vi "Network Error Core.vi"(8 "error in (no error)":errorcluster, 10 "String to Append":string, 11 "Error":T1) -> (0 "error out":errorcluster)   [LabVIEW 2021, in "Networking_CIF_U.lvlib"]
uses:
  Networking_CIF_U.lvlib
  Typedef/Errors.ctl
  Errors/Errors_CIF_U.lvlib
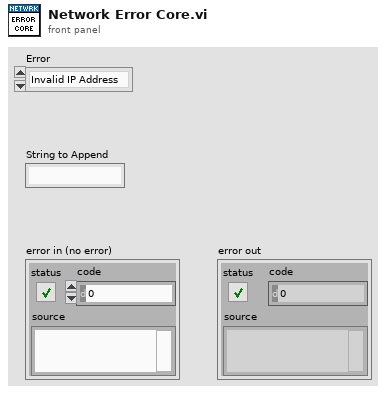
[diagram p1: front panel]
types:
  T1 = typedef "Networking_CIF_U.lvlib/Errors.ctl" = enum16{"Invalid IP Address", "No Subnet Match Found", "Error Finding Port", "No Ping Response", "Nettools Needed", "Error Checking Port"}
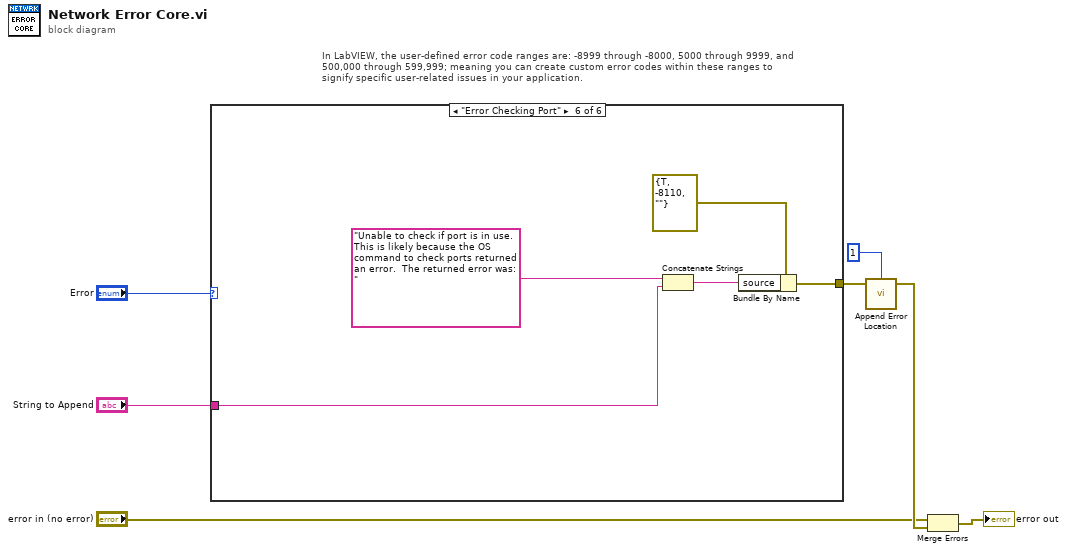
[diagram p0: block diagram]
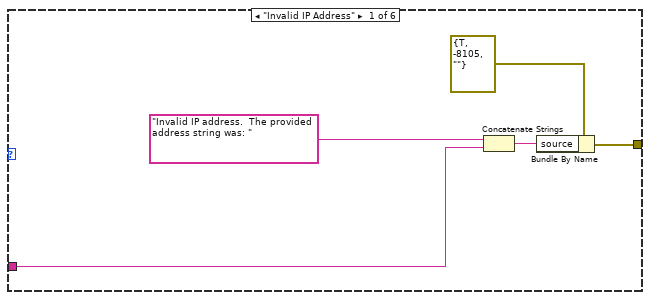
[diagram p2: hidden frame]
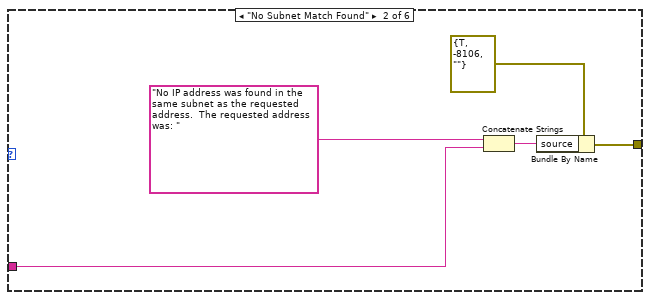
[diagram p3: hidden frame]
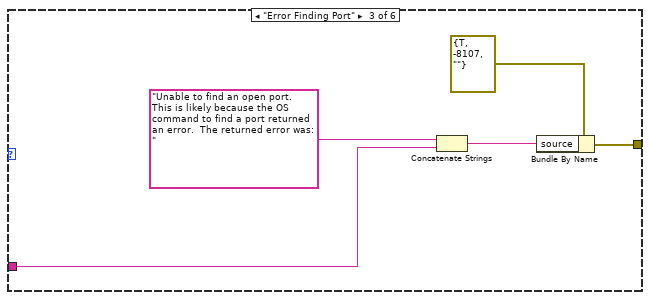
[diagram p4: hidden frame]
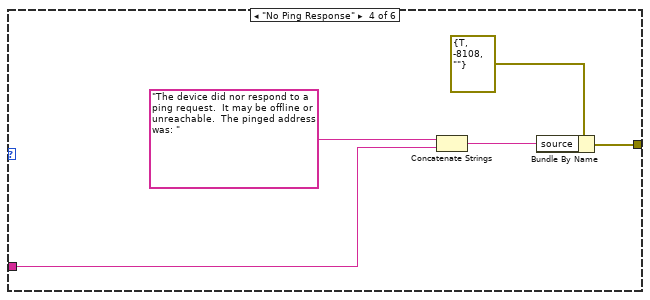
[diagram p5: hidden frame]
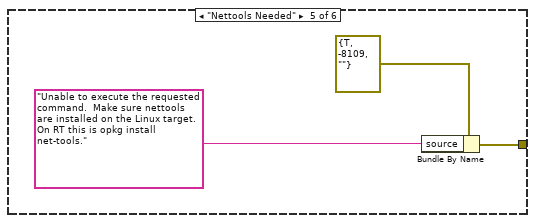
[diagram p6: hidden frame]
diagram:
  # "In LabVIEW, the user-defined error code ranges are: -8999 through -8000, 5000 through 9999, and 500,000 through 599,999; meaning you can create custom error codes within these ranges to signify specific user-related issues in your application."
  n1 = case shown="\"Error Checking Port\"" "Error" {
    tunnel: "String to Append" -> [w9 w14 w18 w23 _ w31]
    tunnel: [w11 w16 w21 w26 w29 w34] -> w6
    frame "Invalid IP Address" {
      n2 = Concatenate Strings("Invalid IP address.  The provided address string was: " ("source"), w9) -> (w8:string)
      n3 = Bundle By Name(cluster=errorcluster {"status"=TRUE, "code"=-8105, "source"=""} ("Invalid ID"), "source"=w8) -> (w11:errorcluster)
    }
    frame "No Subnet Match Found" {
      n4 = Concatenate Strings("No IP address was found in the same subnet as the requested address.  The requested address was: " ("source"), w14) -> (w13:string)
      n5 = Bundle By Name(cluster=errorcluster {"status"=TRUE, "code"=-8106, "source"=""} ("Invalid ID"), "source"=w13) -> (w16:errorcluster)
    }
    frame "Error Finding Port" {
      n6 = Concatenate Strings("Unable to find an open port.  This is likely because the OS command to find a port returned an error.  The returned error was: " ("source"), w18) -> (w19:string)
      n7 = Bundle By Name(cluster=errorcluster {"status"=TRUE, "code"=-8107, "source"=""} ("Invalid ID"), "source"=w19) -> (w21:errorcluster)
    }
    frame "No Ping Response" {
      n8 = Concatenate Strings("The device did nor respond to a ping request.  It may be offline or unreachable.  The pinged address was: " ("source"), w23) -> (w24:string)
      n9 = Bundle By Name(cluster=errorcluster {"status"=TRUE, "code"=-8108, "source"=""} ("Invalid ID"), "source"=w24) -> (w26:errorcluster)
    }
    frame "Nettools Needed" {
      n10 = Bundle By Name(cluster=errorcluster {"status"=TRUE, "code"=-8109, "source"=""} ("Invalid ID"), "source"="Unable to execute the requested command.  Make sure nettools are installed on the Linux target.   On RT this is opkg install net-tools.") -> (w29:errorcluster)
    }
    frame "Error Checking Port" {
      n11 = Concatenate Strings("Unable to check if port is in use.  This is likely because the OS command to check ports returned an error.  The returned error was: " ("source"), w31) -> (w32:string)
      n12 = Bundle By Name(cluster=errorcluster {"status"=TRUE, "code"=-8110, "source"=""} ("Invalid ID"), "source"=w32) -> (w34:errorcluster)
    }
  }
  n13 = call "Append Error Location.vi"("error in (no error)"=w6, "Chain Depth"=1) -> ("error out"=w7:errorcluster)  [unwired: 3 in]
  n14 = Merge Errors("error in (no error)", w7) -> (→"error out":errorcluster)
